vi "PythonValue.vi"(6 "add self":bool, 8 "error in":errorcluster, 11 "ControlTerminal in":refnum<class "ControlTerminal.lvclass">) -> (0 "error out":errorcluster, 3 "ControlTerminal out":refnum<class "ControlTerminal.lvclass">, 5 "value":string)   [LabVIEW 2014, in "Raspberry Pi Compatible Compiler for LabVIEW.lvlib" / "ControlTerminal.lvclass"]
uses:
  ControlTerminal.lvclass
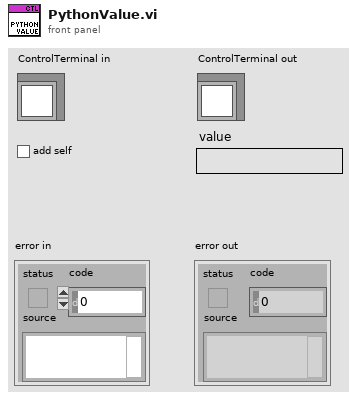
[diagram p1: front panel]
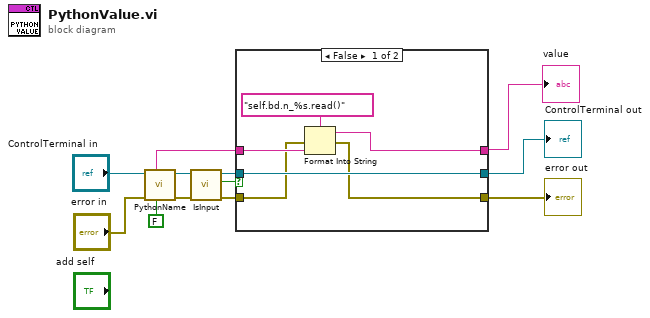
[diagram p0: block diagram]
diagram:
  n1 = call-dynamic "PythonName.vi"("add self"=FALSE, "error in"="error in", "Terminal in"="ControlTerminal in") -> ("error out"=w10:errorcluster, "Terminal out"=w9:refnum<class "ControlTerminal.lvclass">, "UID"=w1:string)  [unwired: 5 in, 1 out]
  n2 = call-dynamic "IsInput.vi"("error in"=w10, "ControlTerminal in"=w9) -> ("error out"=w7:errorcluster, "input"=w8:bool, "ControlTerminal out"=w6:refnum<class "ControlTerminal.lvclass">)  [unwired: 5 in]
  n3 = case shown="False" w8 {
    tunnel: w1 -> [w18 w20]
    tunnel: w7 -> [w15 w21]
    tunnel: w6 -> [w16 w19]
    tunnel: [w16 w19] -> w3
    tunnel: [w14 w21] -> w4
    tunnel: [w13 w20] -> w2
    frame False {
      n4 = Format Into String(format string="self.bd.n_%s.read()", error in=w15, w18) -> (resulting string=w13:string, error out=w14:errorcluster)  [unwired: 1 in]
    }
    frame True {
    }
  }
  "error out" <- w4
  "ControlTerminal out" <- w3
  "value" <- w2
